vi "generate_galvo_voltages_from_fifo.vi"(0 "resonant trigger":bool, 1 "tracking":bool, 5 "counter cluster in":T5, 7 "tracking settings":T1, 9 "scan specification":T4, 11 "scanning":bool, 12 "x-y phase shift (*2^16/2*pi)":u16=16384) -> (3 "update tracking?":T3, 4 "DAC voltages":T6 {"pockels" max=4095 step=1; "y" max=4095 step=1; "x" max=4095 step=1}, 6 "counter cluster out":T5, 10 "fly-back acquisition phase?":bool, 13 "trigger diagnostics":T2, 14 "counting photons?":bool, 15 "acquire?":bool)   [LabVIEW 2010]
uses:
  common_typedefs/DAC_voltage_tagResonantr.ctl
  counter_cluster_tagResonant.ctl
  scan_specification_tagResonant.ctl
  FPGA tracking/polar tracking settings.ctl
  <vilib>/rvi/DataTransferAndStorage/Container/XNode/niFpgaContainer.xnode
  <vilib>/rvi/DataTransferAndStorage/Container/Common/niFpgaContainerMethod.ctl
  <vilib>/rvi/DataTransferAndStorage/Container/Common/niFpgaTransferTypeControl.ctl
  <vilib>/rvi/Analysis/common/FxpNativeNode/niFpgaFxpNative.xnode
  <vilib>/rvi/interface/RandomDataEmulation/nirviRandomDataFPGAFIFO.vi
  <vilib>/rvi/interface/RandomDataEmulation/niFpgaRandomDataHandleErrors.vi
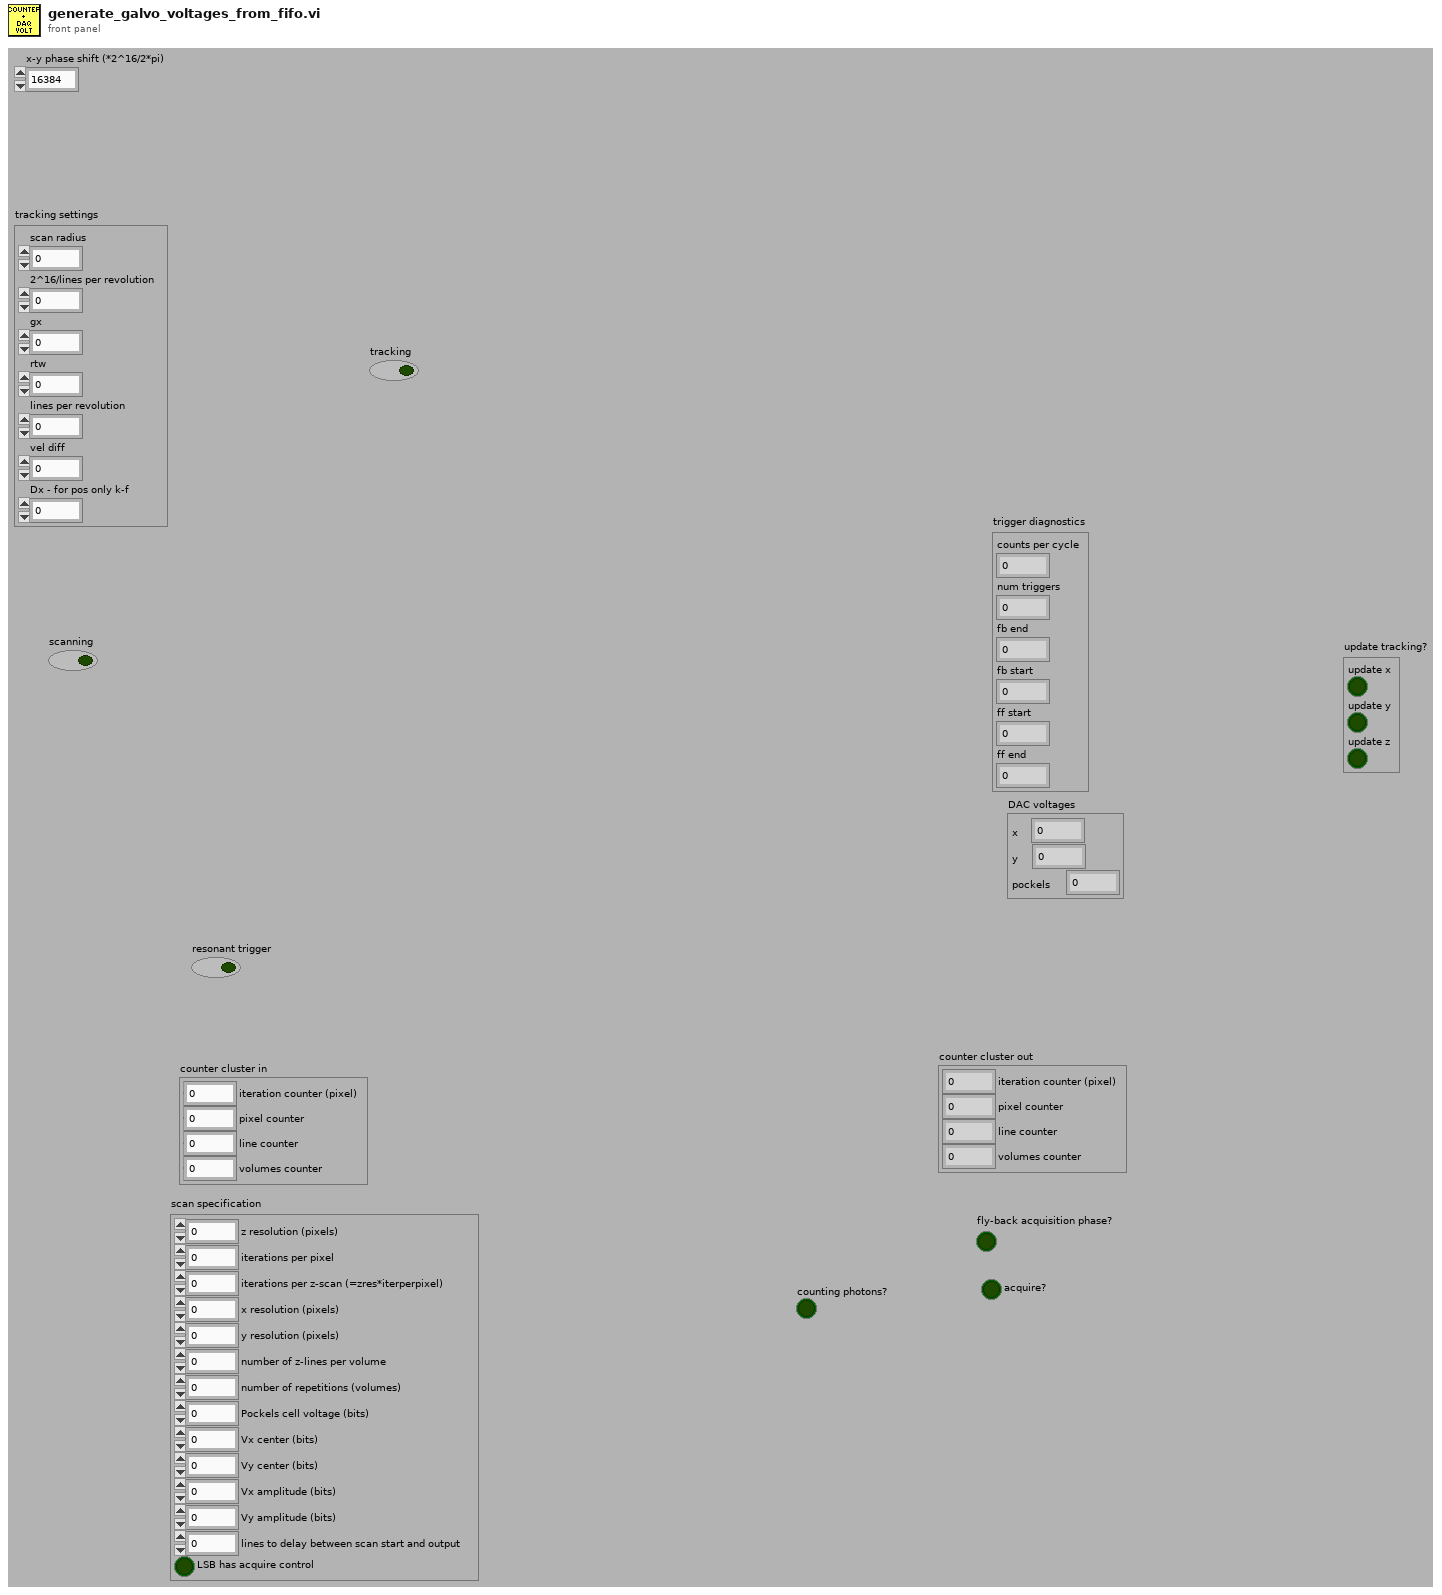
[diagram p1: front panel]
types:
  T1 = typedef "polar tracking settings.ctl" = cluster{"scan radius":u16, "2^16/lines per revolution":u16, "gx":fxp<+,16,8>, "rtw":fxp<+,16,26>, "lines per revolution":u8, "vel diff":fxp<+,24,-22>, "Dx - for pos only k-f":fxp<+,32,19>}
  T2 = cluster{"counts per cycle":u16, "num triggers":u32, "fb end":u16, "fb start":u16, "ff start":u16, "ff end":u16}
  T3 = cluster{"update x":bool, "update y":bool, "update z":bool}
  T4 = typedef "scan_specification_tagResonant.ctl" = cluster{"z resolution (pixels)":u16, "iterations per pixel":u16, "iterations per z-scan (=zres*iterperpixel)":u16, "x resolution (pixels)":u16, "y resolution (pixels)":u16, "number of z-lines per volume":u16, "number of repetitions (volumes)":i32, "Pockels cell voltage (bits)":i16, "Vx center (bits)":i16, "Vy center (bits)":i16, "Vx amplitude (bits)":i16, "Vy amplitude (bits)":i16, "lines to delay between scan start and output":u16, "LSB has acquire control":bool}
  T5 = typedef "counter_cluster_tagResonant.ctl" = cluster{"iteration counter (pixel)":u16, "pixel counter":u16, "line counter":i16, "volumes counter":u16}
  T6 = typedef "DAC_voltage_tagResonantr.ctl" = cluster{"x":i16, "y":i16, "pockels":i16}
  T7 = typedef "niFpgaContainerMethod.ctl" = enum16{"<none>", "write", "read", "clear", "getNumberOfElementsToWrite", "getNumberOfElementsToRead", "enable", "disable", "flushAndDisable", "getStreamState", "readA", "readB", "dramWrite", "dramWriteWithByteEnables", "dramRequestData", "dramRetrieveData"}
  T8 = typedef "niFpgaTransferTypeControl.ctl" = enum16{"Target-Scoped", "Host to Target - DMA", "Target to Host - DMA", "Peer to Peer Reader", "Peer to Peer Writer", "Bidirectional"}
  T9 = cluster{"crossing":bool, "crossing":bool, "crossing":bool}
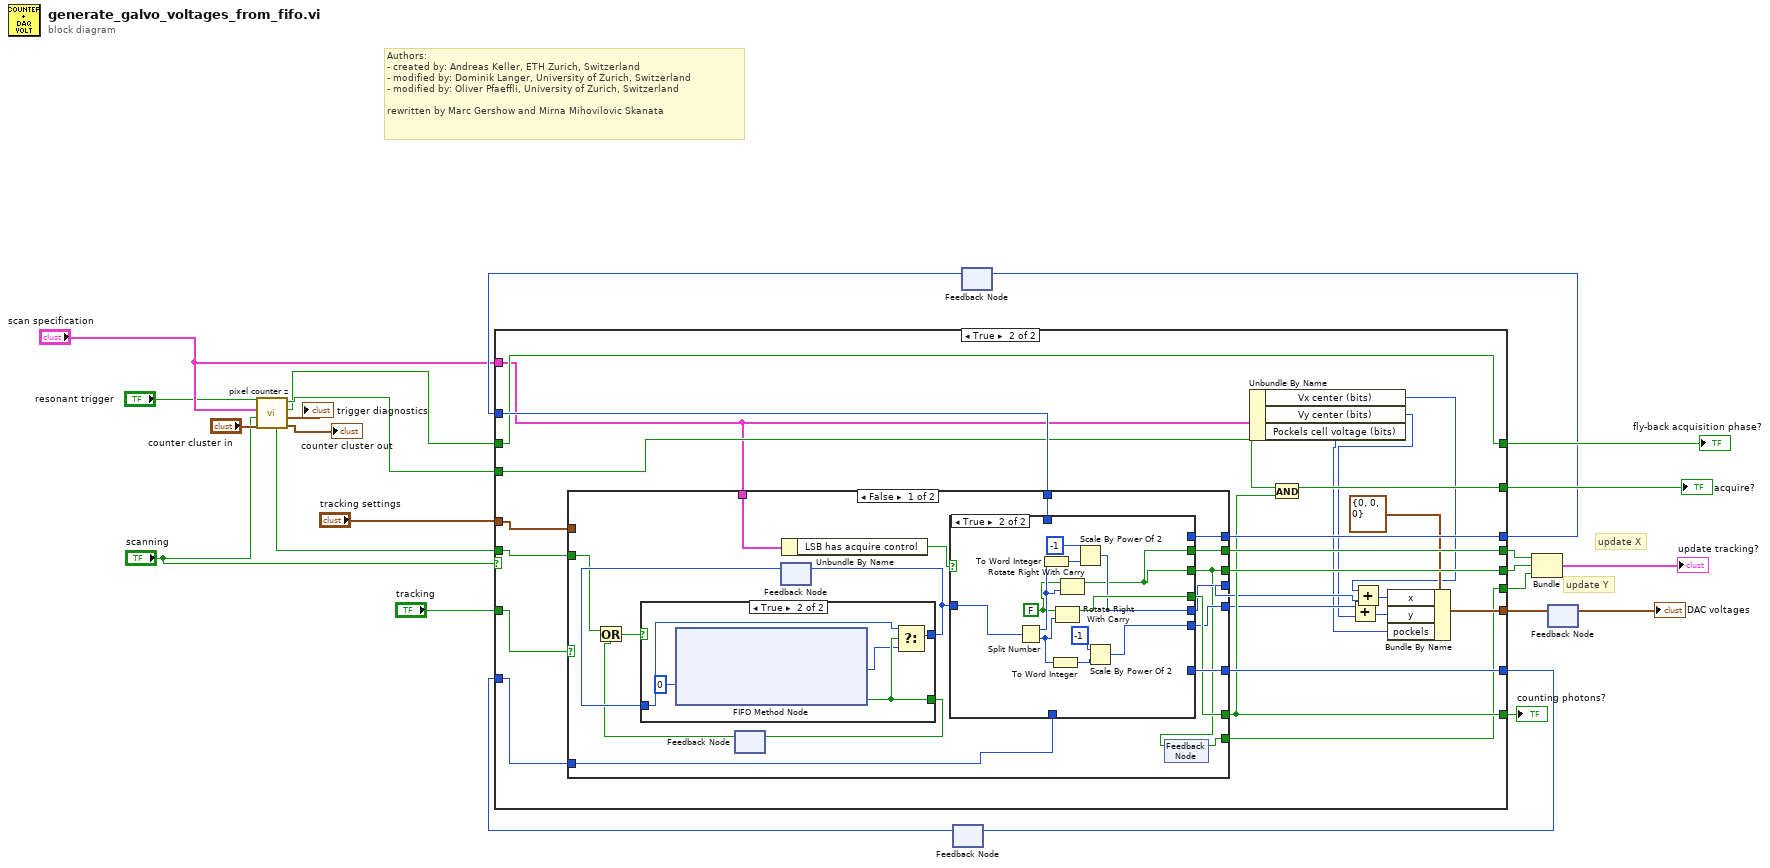
[diagram p0: block diagram]
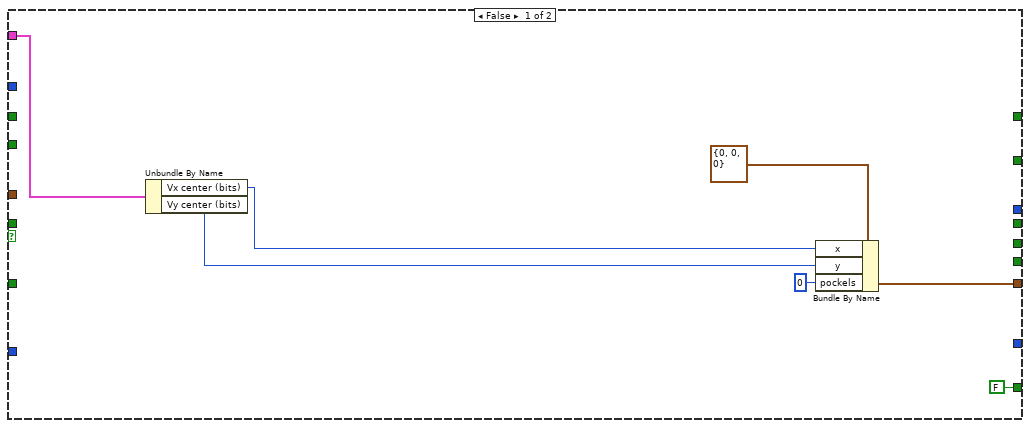
[diagram p2: hidden frame]
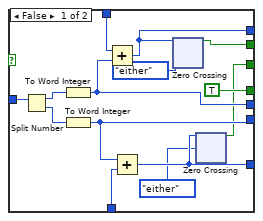
[diagram p3: hidden frame]
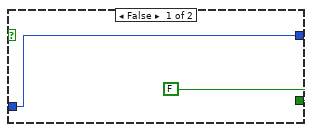
[diagram p4: hidden frame]
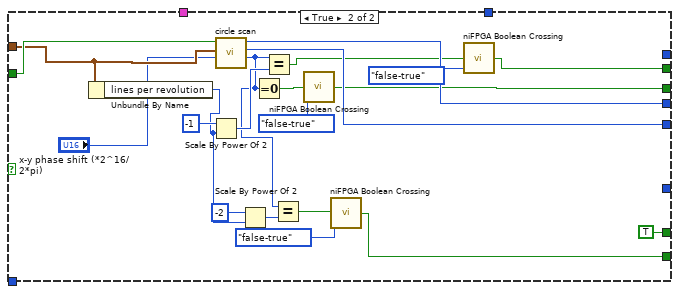
[diagram p5: hidden frame]
diagram:
  # "update Y"
  # "update X"
  # "Authors: \n- created by: Andreas Keller, ETH Zurich, Switzerland\n- modified by: Dominik Langer, University of Zurich, Switzerland\n- modified by: Oliver Pfaeffli, University of Zurich, Switzerland\n\nrewritten by Marc Gershow and Mirna Mihovilovic Skanata"
  n1 = call "pixel counter z.vi"("counter cluster in"="counter cluster in", "scanning"="scanning", "scan specification"="scan specification", "tag lens trigger"="resonant trigger") -> ("counter cluster out"=→"counter cluster out":T5, "trigger diagnostics"=→"trigger diagnostics":T2, "fly back"=w6:bool, "acquire"=w7:bool, "new line"=w8:bool)  [unwired: 3 in]
  n2 = feedback #1() -> (w20:i16)  [unwired: 1 in]
  n3 = feedback #2() -> (w18:i16)  [unwired: 1 in]
  n4 = case shown="True" "scanning" {
    tunnel: [w26 w55] -> w24
    tunnel: [_ w45] -> w23
    tunnel: [_ w48] -> w22
    tunnel: [_ w54] -> w19
    tunnel: [_ w53] -> w21
    tunnel: w20 -> [_ w51]
    tunnel: w18 -> [_ w52]
    tunnel: [_ w50] -> w15
    tunnel: [_ w49] -> w16
    tunnel: [FALSE ("lsb carry out") w47] -> w17
    tunnel: "scan specification" -> [w29 w44]
    tunnel: w8 -> [_ w43]
    tunnel: w7 -> [_ w46]
    tunnel: w6 -> [_ w45]
    tunnel: [_ w32] -> w4
    tunnel: "tracking" -> [_ w34]
    tunnel: "tracking settings" -> [_ w33]
    frame False {
      n5 = Unbundle By Name(w29) -> ("Vx center (bits)"=w28:i16, "Vy center (bits)"=w27:i16)
      n6 = Bundle By Name(cluster=T6 {"x"=0, "y"=0, "pockels"=0} ("DAC voltage"), "x"=w28, "y"=w27, "pockels"=i16 0) -> (w26:T6)
    }
    frame True {
      n7 = case shown="False" w34 {
        tunnel: [w73 _] -> w54
        tunnel: [w72 _] -> w53
        tunnel: w52 -> [w71 _]
        tunnel: w51 -> [w70 _]
        tunnel: [w69 w176] -> w50
        tunnel: [w57 w179] -> w49
        tunnel: [w68 TRUE ("lsb carry out")] -> w47
        tunnel: w44 -> [w67 _]
        tunnel: w43 -> [w58 w185]
        tunnel: [w60 w188] -> w41
        tunnel: [w59 w187] -> w40
        tunnel: w33 -> [_ w184]
        tunnel: [w56 w169] -> w32
        frame False {
          n8 = feedback #3() -> (w63:bool)  [unwired: 1 in]
          n9 = Or(x=w58, y=w63) -> (x .or. y?=w65:bool)
          n10 = feedback #4() -> (w66:u32)  [unwired: 1 in]
          n11 = case shown="True" w65 {
            tunnel: [w133 w137] -> w61
            tunnel: w66 -> [w133 w134]
            tunnel: [FALSE ("Timed Out?") w136] -> w64
            frame False {
            }
            frame True {
              n12 = xnode ("FIFO Method Node")("Timeout"=0) -> ("Element"=w135:u32, "Timed Out?"=w136:bool)  [unwired: 1 in, 1 out]
              n13 = Select(t=w134, s=w136, f=w135) -> (s? t:f=w137:u32)
            }
          }
          n14 = feedback-in #3(w64) -> ()
          n15 = feedback-in #4(w61) -> ()
          n16 = Unbundle By Name(w67) -> ("LSB has acquire control"=w62:bool)
          n17 = case shown="True" w62 {
            tunnel: w61 -> [w86 w131]
            tunnel: [w83 w124] -> w60
            tunnel: [w82 w128] -> w59
            tunnel: [TRUE ("lsb carry out") w126] -> w68
            tunnel: [w74 w120] -> w57
            tunnel: [w77 w120] -> w69
            tunnel: [w79 _] -> w73
            tunnel: [w76 _] -> w72
            tunnel: w71 -> [w81 _]
            tunnel: w70 -> [w80 _]
            frame False {
              n18 = Split Number(x=w86) -> (hi(x)=w85:u16, lo(x)=w84:u16)
              n19 = To Word Integer(number=w85) -> (16bit integer=w83:i16)
              n20 = To Word Integer(number=w84) -> (16bit integer=w82:i16)
              n21 = Add(x=w81, y=w83) -> (x+y=w79:i16)
              n22 = Add(x=w82, y=w80) -> (x+y=w76:i16)
              n23 = xnode ("Zero Crossing")("direction"=enum8{"either", "minus-plus", "plus-minus"}."either", "input"=w79) -> ("crossing"=w77:bool)  [unwired: 1 in]
              n24 = xnode ("Zero Crossing")("direction"=enum8{"either", "minus-plus", "plus-minus"}."either", "input"=w76) -> ("crossing"=w74:bool)  [unwired: 1 in]
            }
            frame True {
              w121 = FALSE ("carry")
              n25 = Split Number(x=w131) -> (hi(x)=w122:u16, lo(x)=w130:u16)
              n26 = To Word Integer(number=w122) -> (16bit integer=w125:i16)
              n27 = To Word Integer(number=w130) -> (16bit integer=w127:i16)
              n28 = Rotate Right With Carry(2:w130, 3:w121) -> (1:w126:bool)  [unwired: 1 out]
              n29 = Rotate Right With Carry(2:w122, 3:w121) -> (1:w120:bool)  [unwired: 1 out]
              n30 = Scale By Power Of 2(n=-1, x=w125) -> (x*2^n=w124:i16)
              n31 = Scale By Power Of 2(n=-1, x=w127) -> (x*2^n=w128:i16)
            }
          }
          n32 = feedback-in #5(w57) -> ()
          n33 = feedback #5() -> (w56:bool)  [unwired: 1 in]
        }
        frame True {
          n34 = Unbundle By Name(w184) -> ("lines per revolution"=w173:u8)
          n35 = Scale By Power Of 2(n=-1, x=w173) -> (x*2^n=w182:u8)
          n36 = call "circle scan.vi"("x-y phase shift (*2^16/2*pi)"="x-y phase shift (*2^16/2*pi)", "tracking settings"=w184, "new line"=w185) -> ("line counter"=w174:u8, "y value"=w187:i16, "x value"=w188:i16)  [unwired: 6 in]
          n37 = Scale By Power Of 2(n=-2, x=w173) -> (x*2^n=w172:u8)
          n38 = Equal To 0?(x=w174) -> (x = 0?=w181:bool)
          n39 = Equal?(x=w174, y=w182) -> (x = y?=w177:bool)
          n40 = Equal?(x=w174, y=w172) -> (x = y?=w170:bool)
          n41 = call <vilib>:"niFPGA Boolean Crossing.vi"("input"=w181, "direction"=enum8{"either", "false-true", "true-false"}."false-true") -> ("crossing"=w179:bool)  [unwired: 7 in]
          n42 = call <vilib>:"niFPGA Boolean Crossing.vi"("input"=w170, "direction"=enum8{"either", "false-true", "true-false"}."false-true") -> ("crossing"=w169:bool)  [unwired: 7 in]
          n43 = call <vilib>:"niFPGA Boolean Crossing.vi"("input"=w177, "direction"=enum8{"either", "false-true", "true-false"}."false-true") -> ("crossing"=w176:bool)  [unwired: 7 in]
        }
      }
      n44 = Unbundle By Name(w44) -> ("Vx center (bits)"=w38:i16, "Vy center (bits)"=w36:i16, "Pockels cell voltage (bits)"=w35:i16)
      n45 = And(x=w46, y=w47) -> (x .and. y?=w48:bool)
      n46 = Add(x=w40, y=w36) -> (x+y=w37:i16)
      n47 = Add(x=w38, y=w41) -> (x+y=w39:i16)
      n48 = Bundle By Name(cluster=T6 {"x"=0, "y"=0, "pockels"=0} ("DAC voltage"), "x"=w39, "y"=w37, "pockels"=w35) -> (w55:T6)
    }
  }
  "acquire?" <- w22
  "fly-back acquisition phase?" <- w23
  "counting photons?" <- w17
  n49 = feedback-in #1(w21) -> ()
  n50 = feedback-in #2(w19) -> ()
  n51 = Bundle("crossing"=w15, "crossing"=w16, "crossing"=w4) -> (→"update tracking?":T9)  [unwired: 1 in]
  n52 = feedback-in #6(w24) -> ()
  n53 = feedback #6() -> (→"DAC voltages":T6)  [unwired: 1 in]
